vi "load.vi"(8 "error in (no error)":errorcluster, 10 "Path":path, 11 "RoiCollection in":refnum<class "RoiCollection.lvclass">) -> (0 "error out":errorcluster, 3 "RoiCollection out":refnum<class "RoiCollection.lvclass">)   [LabVIEW 2010, in "RoiCollection.lvclass"]
uses:
  RoiCollection.lvclass
  <vilib>/regexp/Match Regular Expression.xnode
  RoiGeneric/RoiGeneric.lvclass
  RoiEllipsoid/RoiEllipsoid.lvclass
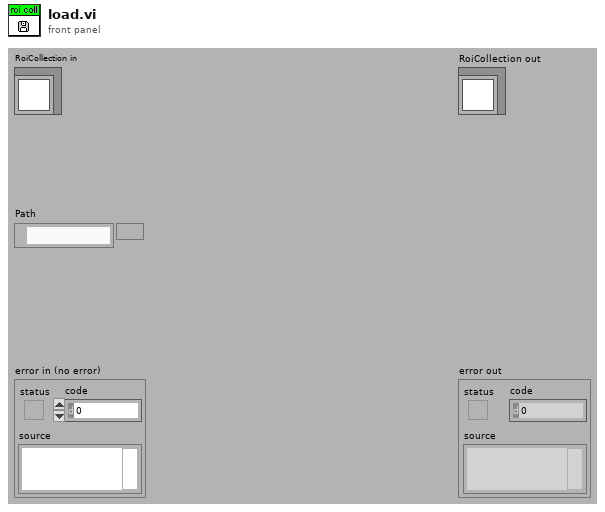
[diagram p1: front panel]
types:
  T1 = enum16{"open", "replace", "create", "open or create", "replace or create", "replace or create with confirmation"}
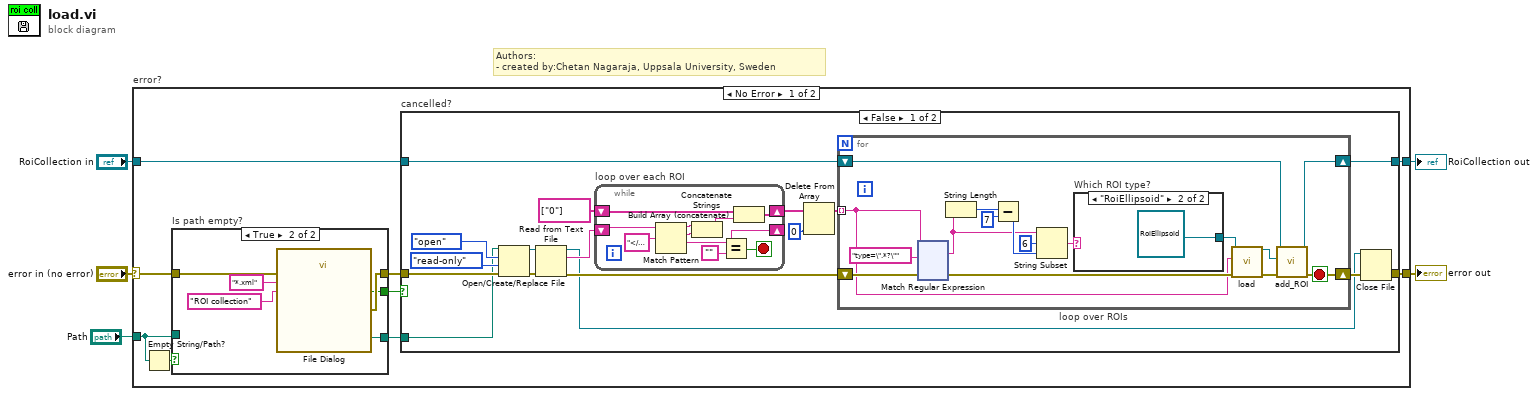
[diagram p0: block diagram]
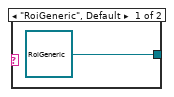
[diagram p2: hidden frame]
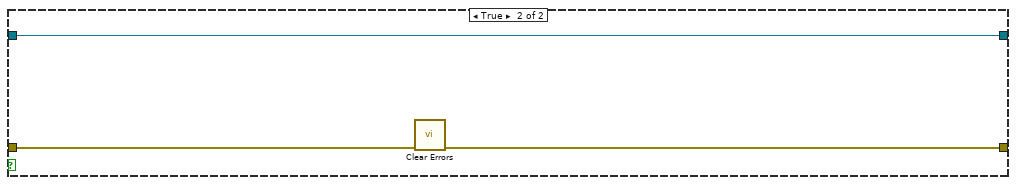
[diagram p3: hidden frame]
diagram:
  # "Authors: \n- created by:Chetan Nagaraja, Uppsala University, Sweden"
  n1 = case "error?" shown="No Error" "error in (no error)" {
    selector: "error in (no error)" -> [w11 w182]
    tunnel: [w14 w183] -> w3
    tunnel: "RoiCollection in" -> [w13 w183]
    tunnel: "Path" -> [w7 _]
    tunnel: [w12 w182] -> w1
    frame No Error {
      n2 = Empty String/Path?(string/path=w7) -> (empty?=w9:bool)
      n3 = case "Is path empty?" shown="True" w9 {
        tunnel: w11 -> [w175 w181]
        tunnel: [w175 w180] -> w10
        tunnel: [w174 w179] -> w8
        tunnel: w7 -> [w174 _]
        tunnel: [_ w178] -> w6
        frame False {
        }
        frame True {
          n4 = call "File Dialog"("error in"=w181, "pattern (all files)"="*.xml", "pattern label"="ROI collection") -> ("selected path"=w179:path, "cancelled"=w178:bool, "error out"=w180:errorcluster)  [unwired: 9 in, 1 out]
        }
      }
      n5 = case "cancelled?" shown="False" w6 {
        tunnel: [w16 w173] -> w14
        tunnel: w13 -> [w17 w173]
        tunnel: [w28 w171] -> w12
        tunnel: w10 -> [w27 w172]
        tunnel: w8 -> [w26 _]
        frame False {
          n6 = Open/Create/Replace File(file path (use dialog)=w26, error in=w27, operation (0:open)=T1."open", access (0:read/write)=enum16{"read/write", "read-only", "write-only"}."read-only") -> (refnum out=w23:refnum<file>, error out=w25:errorcluster)  [unwired: 2 in, 1 out]
          n7 = Read from Text File(file (use dialog)=w23, error in=w25) -> (refnum out=w15:refnum<file>, text=w19:string, error out=w24:errorcluster)  [unwired: 2 in, 1 out]
          n8 = while "loop over each ROI" {
            shift-right: [w32] -> _
            shift-left: w19 -> [w38]
            shift-right: [w39] -> w21
            shift-left: string[] ["0"] -> [w40]
            stop <- w36 stop-if-true
            n9 = Match Pattern(string=w38, regular expression="</RoiGeneric>") -> (before substring=w35:string, match substring=w34:string, after substring=w32:string)  [unwired: 1 in, 1 out]
            n10 = Concatenate Strings(w35, w34) -> (w33:string)
            n11 = Equal?(x=w32, y="") -> (x = y?=w36:bool)
            n12 = Build Array (concatenate)(w40, w33) -> (w39:string[])
          }
          n13 = Delete From Array(array=w21, index=0) -> (array with subset deleted=w18:string[])  [unwired: 1 in, 1 out]
          n14 = for "loop over ROIs" {
            shift-right: [w54] -> w29
            shift-left: w24 -> [w52]
            tunnel: w18 -> [w43] mode=indexing
            shift-right: [w56] -> w16
            shift-left: w17 -> [w57]
            stop <- w54 stop-if-true
            n15 = xnode "Match Regular Expression"("input string"=w43, "regular expression"="type=\".*?\"", "error in"=w52) -> ("whole match"=w42:string, "error out"=w51:errorcluster)  [unwired: 3 in, 3 out]
            n16 = String Length(string=w42) -> (length=w48:i32)
            n17 = Subtract(x=w48, y=7) -> (x-y=w46:i32)
            n18 = String Subset(string=w42, offset (0)=6, length (rest)=w46) -> (substring=w45:string)
            n19 = case "Which ROI type?" shown="\"RoiEllipsoid\"" w45 {
              tunnel: [refnum<class "RoiGeneric.lvclass"> refnum ("RoiGeneric.lvclass") refnum<class "RoiEllipsoid.lvclass"> refnum ("RoiEllipsoid.lvclass")] -> w44
              frame "RoiGeneric", Default {
              }
              frame "RoiEllipsoid" {
              }
            }
            n20 = call-dynamic "load.vi"("error in (no error)"=w51, "XML String"=w43, "RoiGeneric in"=w44) -> ("error out"=w55:errorcluster, "RoiGeneric out"=w53:refnum<class "RoiGeneric.lvclass">)  [unwired: 7 in]
            n21 = call "add_ROI.vi"("error in (no error)"=w55, "roi"=w53, "RoiCollection in"=w57) -> ("error out"=w54:errorcluster, "RoiCollection out"=w56:refnum<class "RoiCollection.lvclass">)  [unwired: 7 in]
          }
          n22 = Close File(2:w29, 3:w15) -> (0:w28:errorcluster)  [unwired: 1 out]
        }
        frame True {
          n23 = call <vilib>:"Clear Errors.vi"("error in (no error)"=w172) -> ("error out"=w171:errorcluster)  [unwired: 6 in]
        }
      }
    }
    frame Error {
    }
  }
  "error out" <- w1
  "RoiCollection out" <- w3
